vi "Execute.vi"(7 "user event in":refnum<user-event>, 8 "Advanced Waveform In":refnum<class "Advanced Waveform.lvclass">, 9 "Gen Sine in":refnum<class "Gen Sine.lvclass">, 10 "Command Queue":refnum<queue>, 11 "error in (no error)":errorcluster) -> (0 "Advanced Waveform Out":refnum<class "Advanced Waveform.lvclass">, 1 "Gen Sine out":refnum<class "Gen Sine.lvclass">, 2 "Stop":bool, 3 "error out":errorcluster)   [LabVIEW 2011, in "Gen Sine.lvclass"]
uses:
  Gen Sine.lvclass
  Advanced Waveform Class/Advanced Waveform.lvclass
  Message.lvclass
  Display Message/Display Message.lvclass
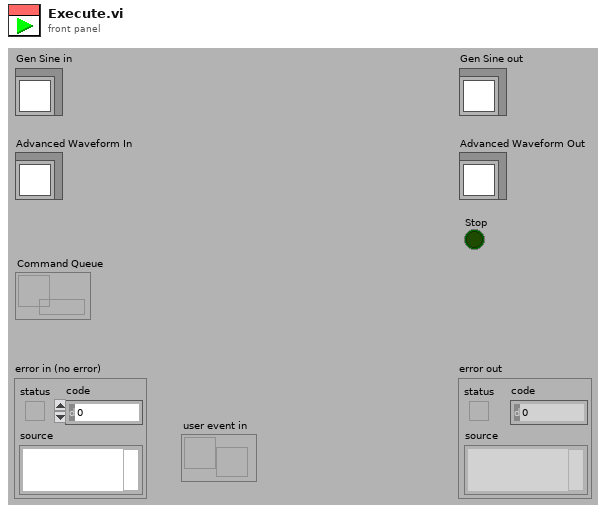
[diagram p1: front panel]
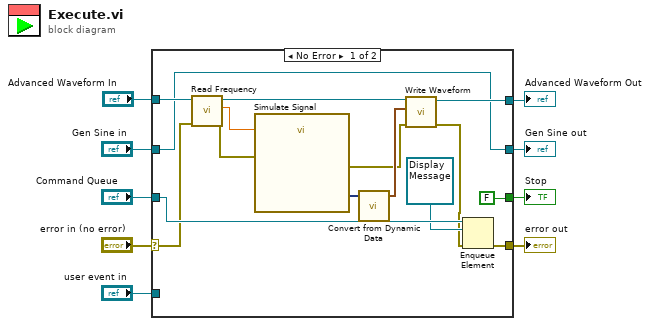
[diagram p0: block diagram]
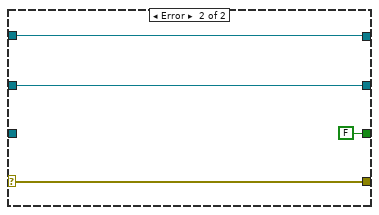
[diagram p2: hidden frame]
diagram:
  n1 = case shown="No Error" "error in (no error)" {
    selector: "error in (no error)" -> [w14 w26]
    tunnel: "Advanced Waveform In" -> [w24 w28]
    tunnel: "Gen Sine in" -> [w10 w27]
    tunnel: [w21 w28] -> w6
    tunnel: [w10 w27] -> w5
    tunnel: "Command Queue" -> [w18 _]
    tunnel: [w12 w26] -> w3
    tunnel: "user event in" -> [_ _]
    tunnel: [FALSE FALSE] -> w1
    frame No Error {
      n2 = call-dynamic "Read Frequency.vi"("error in (no error)"=w14, "Waveform in"=w24) -> ("error out"=w15:errorcluster, "Frequency"=w23:dbl, "Waveform out"=w22:refnum<class "Advanced Waveform.lvclass">)  [unwired: 7 in]
      n3 = call "Simulate Signal"("Frequency"=w23, "error in (no error)"=w15) -> ("Sine"=w20:dynamicdata, "error out"=w16:errorcluster)  [unwired: 12 in]
      n4 = call "Convert from Dynamic Data"("Dynamic Data Type"=w20) -> ("Waveform"=w19:waveform(dbl))  [unwired: 3 in]
      n5 = call-dynamic "Write Waveform.vi"("error in (no error)"=w16, "Waveform"=w19, "Waveform in"=w22) -> ("error out"=w13:errorcluster, "Waveform out"=w21:refnum<class "Advanced Waveform.lvclass">)  [unwired: 7 in]
      n6 = Enqueue Element(queue=w18, element=refnum<class "Display Message.lvclass"> refnum ("Display Message.lvclass"), error in (no error)=w13) -> (error out=w12:errorcluster)  [unwired: 1 in, 2 out]
    }
    frame Error {
    }
  }
  "error out" <- w3
  "Gen Sine out" <- w5
  "Stop" <- w1
  "Advanced Waveform Out" <- w6
